vi "salProcessorCMD.vi"(8 "error in (no error)":errorcluster, 11 "SALCommunicatorController in":refnum<class "SALCommunicatorController.lvclass">) -> (0 "error out":errorcluster, 3 "SALCommunicatorController out":refnum<class "SALCommunicatorController.lvclass">)   [LabVIEW 2016, in "SALCommunicatorController.lvclass"]
uses:
  SALCommunicatorController.lvclass
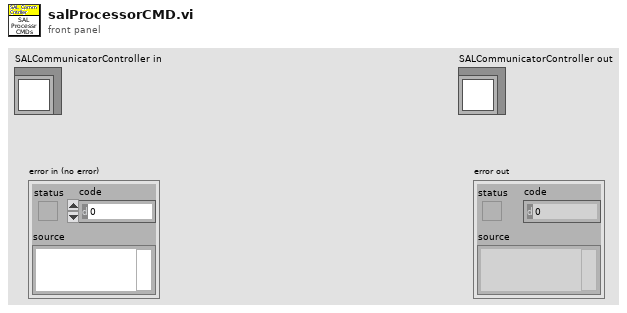
[diagram p1: front panel]
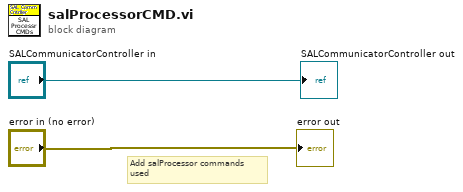
[diagram p0: block diagram]
diagram:
  # "Add salProcessor commands\nused"
  "error out" <- "error in (no error)"
  "SALCommunicatorController out" <- "SALCommunicatorController in"
